vi "PH_SSAC.check Frames.vi"(0 "i ref in":refnum<vi>, 5 "error in":errorcluster) -> (13 "All ok?":bool, 14 "i ref out":refnum<vi>, 15 "x Dimension Main ok?":bool, 16 "y Dimension Main ok?":bool, 17 "x Dimension Background ok?":bool, 18 "y Dimension Background ok?":bool, 19 "error out":errorcluster)   [LabVIEW 2014, in "PH_SSAC.lvlib"]
doc: "This VI checks the image size and whether the size of the main and the background frames fit into it."
uses:
  PH_SSAC.lvlib
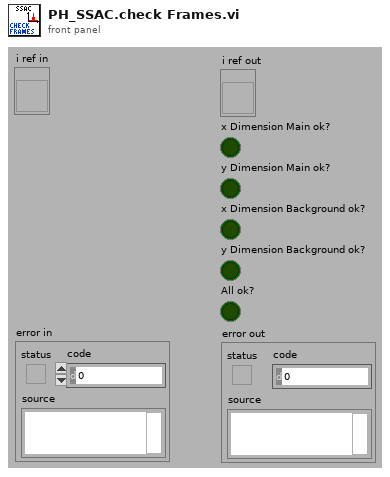
[diagram p1: front panel]
types:
  T1 = typedef "PH_SSAC.lvlib/PH_SSAC.i attribute.ctl" = cluster{"GUI Refs":cluster{"Delete":refnum<vi>, "Global On":refnum<vi>, "Cam Source":refnum<vi>, "Frame Main Signal":refnum<vi>, "Frame Background":refnum<vi>, "dt (Gauss smooth)":refnum<vi>, "Calibration Factor":refnum<vi>, "Background acquire":refnum<vi>, "Threshold":refnum<vi>, "Time evolution of mean pulse duration":refnum<vi>, "Mean Pulse Duration":refnum<vi>, "Main signal":refnum<vi>, "Current Pulse Duration":refnum<vi>, "Processed":refnum<vi>, "Saturation":refnum<vi>, "# for Average":refnum<vi>, "Position":refnum<vi>, "BG Status":refnum<vi>, "Save BG data":refnum<vi>, "Read BG Data":refnum<vi>, "Background Calibration Data":refnum<vi>}, "Images":cluster{"OP Image":T2, "GUI Image":T2, "PSDB Image":T2}, "Global On?":bool, "Frame Main":cluster{"x":u32, "dx":u32, "y":u32, "dy":u32}, "Frame Background":cluster{"x":u32, "dx":u32, "y":u32, "dy":u32}, "dt [fs]":dbl, "Calibration Factor [fs/pixel]":dbl, "Threshold":dbl, "Time evolution of mean pulse duration [fs]":dbl[], "Main Signal":cluster{"Time for Main":dbl[], "Signal":dbl[]}, "Processed":bool, "Current Pulse Duration [fs]":dbl, "# for Average":i32, "Position":i32, "Pulse Durations [fs]":dbl[], "BG":cluster{"Acquire?":bool, "Background Calibration Data":T3, "Save Data":bool}}
  T2 = typedef "IMAQ Image.ctl" = refnum<image>
  T3 = typedef "PH_SSAC.lvlib/PH_SSAC.Background Data.ctl" = cluster{"Date":string, "Time":string, "Frame Main":cluster{"x":u32, "dx":u32, "y":u32, "dy":u32}, "dt [fs]":dbl, "Calibration Factor [fs/pixel]":dbl, "Signal":dbl[], "Frame Background":cluster{"x":u32, "dx":u32, "y":u32, "dy":u32}}
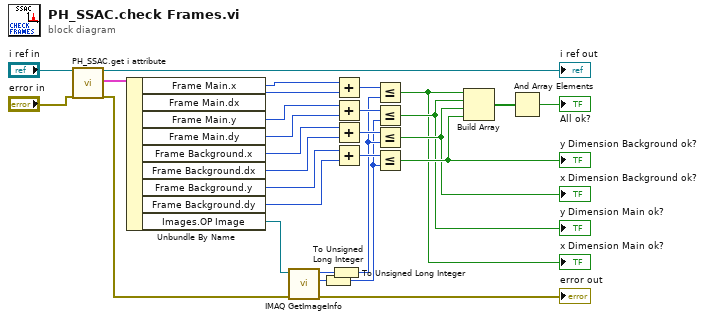
[diagram p0: block diagram]
diagram:
  n1 = call "PH_SSAC.get i attribute.vi"("i ref in"="i ref in", "error in (no error)"="error in") -> ("i ref out"=→"i ref out":refnum<vi>, "i attribute"=w27:T1, "error out"=w25:errorcluster)  [unwired: 15 in]
  n2 = Unbundle By Name(w27) -> ("Frame Main.x"=w20:u32, "Frame Main.dx"=w16:u32, "Frame Main.y"=w19:u32, "Frame Main.dy"=w11:u32, "Frame Background.x"=w23:u32, "Frame Background.dx"=w10:u32, "Frame Background.y"=w24:u32, "Frame Background.dy"=w9:u32, "Images.OP Image"=w26:T2)
  n3 = call "IMAQ GetImageInfo"("error in (no error)"=w25, "Image"=w26) -> ("error out"=→"error out":errorcluster, "Y Resolution"=w14:i32, "X Resolution"=w15:i32)  [unwired: 2 in, 5 out]
  n4 = To Unsigned Long Integer(number=w14) -> (unsigned 32bit integer=w12:u32)
  n5 = To Unsigned Long Integer(number=w15) -> (unsigned 32bit integer=w13:u32)
  n6 = Add(x=w20, y=w16) -> (x+y=w18:u32)
  n7 = Add(x=w19, y=w11) -> (x+y=w17:u32)
  n8 = Add(x=w23, y=w10) -> (x+y=w21:u32)
  n9 = Add(x=w24, y=w9) -> (x+y=w22:u32)
  n10 = Less Or Equal?(x=w18, y=w13) -> (x <= y?=w1:bool)
  "x Dimension Main ok?" <- w1
  n11 = Less Or Equal?(x=w17, y=w12) -> (x <= y?=w2:bool)
  "y Dimension Main ok?" <- w2
  n12 = Less Or Equal?(x=w21, y=w13) -> (x <= y?=w3:bool)
  "x Dimension Background ok?" <- w3
  n13 = Less Or Equal?(x=w22, y=w12) -> (x <= y?=w4:bool)
  "y Dimension Background ok?" <- w4
  n14 = Build Array(w1, w2, w3, w4) -> (w6:bool[])
  n15 = And Array Elements(Boolean array=w6) -> (logical AND=→"All ok?":bool)
